vi "NI VeriStand - Get System Node Channel List.vi"(8 "error in (no error)":errorcluster, 10 "StartNode (\"\")":string, 11 "WorkspaceManager in":T3) -> (0 "error out":errorcluster {"code" format="%.0x"}, 2 "Channels":T1[](array[typedef]), 3 "WorkspaceManager out":T3)   [LabVIEW 2020, in "NI_VS Workspace ExecutionAPI.lvlib"]
doc: "Returns information about all the channels under the specified system node."
uses:
  <vilib>/NI VeriStand/Execution/Workspace/NI_VS Workspace ExecutionAPI.lvlib
  <vilib>/NI VeriStand/Execution/Workspace/WorkspaceAPI.ctl
  NationalInstruments.VeriStand.ClientAPI
  <vilib>/NI VeriStand/Execution/Workspace/NodeInfo.ctl
  <vilib>/NI VeriStand/Execution/Workspace/Waveform Data Type.ctl
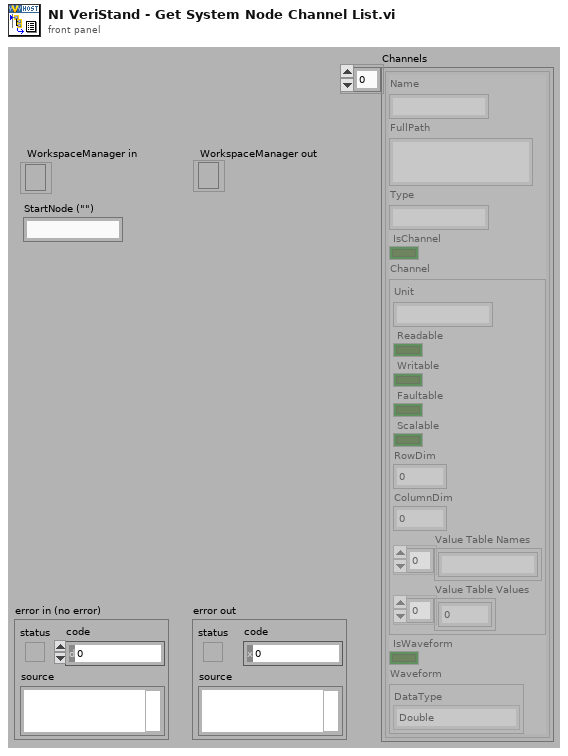
[diagram p1: front panel]
types:
  T1 = typedef "NI_VS Workspace ExecutionAPI.lvlib/NodeInfo.ctl" = cluster{"Name":string, "FullPath":string, "Type":string, "IsChannel":bool, "Channel":cluster{"Unit":string, "Readable":bool, "Writable":bool, "Faultable":bool, "Scalable":bool, "RowDim":u32, "ColumnDim":u32, "Value Table Names":string[], "Value Table Values":dbl[]}, "IsWaveform":bool, "Waveform":cluster{"DataType":T2}}
  T2 = typedef "NI_VS Workspace ExecutionAPI.lvlib/Waveform Data Type.ctl" = enum16{"Double", "ComplexDouble"}
  T3 = typedef "NI_VS Workspace ExecutionAPI.lvlib/WorkspaceAPI.ctl" = refnum<k24>
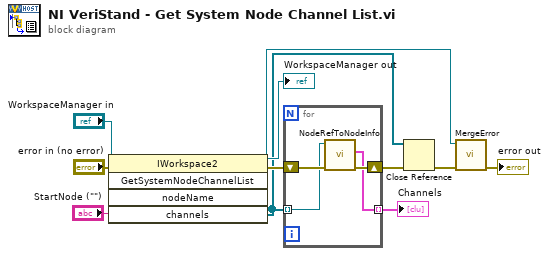
[diagram p0: block diagram]
diagram:
  n1 = invoke class="IWorkspace2" method="GetSystemNodeChannelList"(reference="WorkspaceManager in", error in="error in (no error)", "nodeName"="StartNode (\"\")") -> (reference out=→"WorkspaceManager out":T3, error out=w5:errorcluster, "GetSystemNodeChannelList"=w4:refnum<k24>, "channels"=w1:refnum<k24>[])  [unwired: 2 in, 1 out]
  n2 = for {
    shift-right: [w14] -> w7
    shift-left: w5 -> [w15]
    tunnel: [w13] -> w3 mode=indexing
    tunnel: w1 -> [w12] mode=indexing
    n3 = call <vilib>:"NodeRefToNodeInfo.vi"("error in (no error)"=w15, "Node"=w12) -> ("error out"=w14:errorcluster, "NodeInfo"=w13:T1)  [unwired: 8 out]
  }
  "Channels" <- w3
  n4 = Close Reference(reference=w1, error in (no error)=w7) -> (error out=w6:errorcluster)
  n5 = call <vilib>:"MergeError.vi"("error in (no error)"=w6, "Error"=w4) -> ("error out"=→"error out":errorcluster)  [unwired: 9 out]
